vi "Emi EEp.vi"(6 "Num Emi In":u16, 7 "Num Image":u8, 8 "entrée d'erreur":errorcluster caption="entrée d'erreur (pas d'erreur)", 9 "Emi Image EEp":bool, 10 "Matrix en entrée":u8[](array[numeric]), 11 "X-CAN en entrée":refnum<class "X-CAN.lvclass">) -> (0 "sortie d'erreur":errorcluster, 1 "Etat Emi EEp":u16(slide) scale=0.0..512.0, 3 "X-CAN en sortie":refnum<class "X-CAN.lvclass">, 4 "Num Emi Out":u16)   [LabVIEW 2014]
uses:
  <vilib>/Stratom, Inc/X-CAN for myRIO (API)/X-CAN Class/X-CAN.lvclass
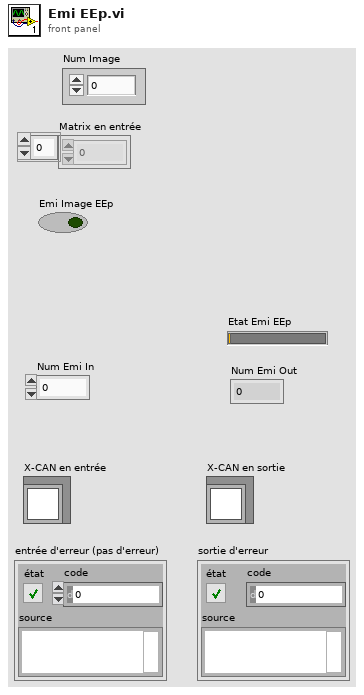
[diagram p1: front panel]
types:
  T1 = cluster{"ID trame":u32, bool, bool, i32[], "seconds since 1Jan1904":timestamp}
  T2 = cluster{"ID trame":u32, bool, bool, u8[], "seconds since 1Jan1904":timestamp}
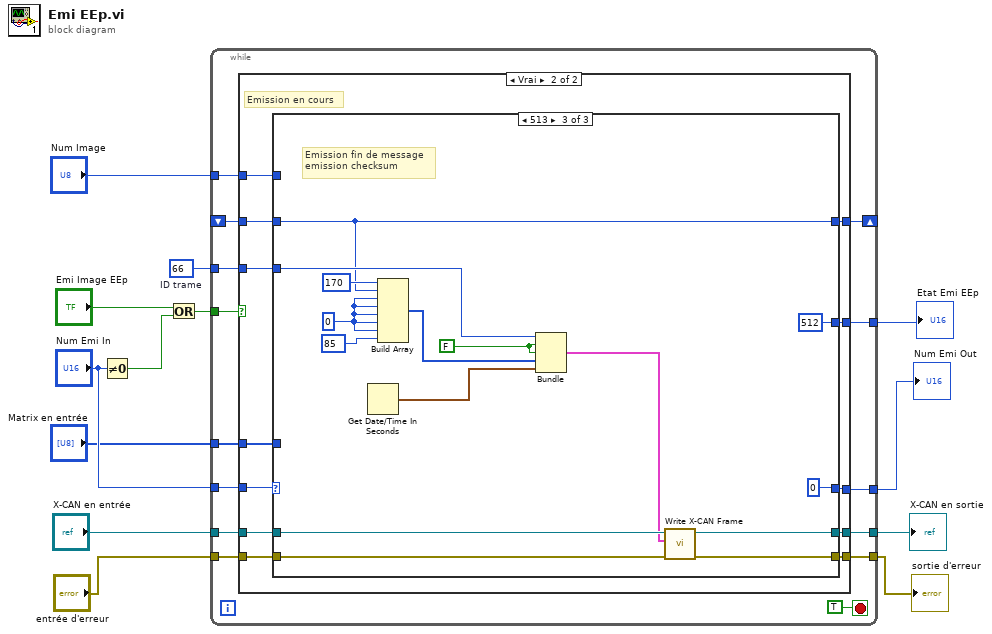
[diagram p0: block diagram]
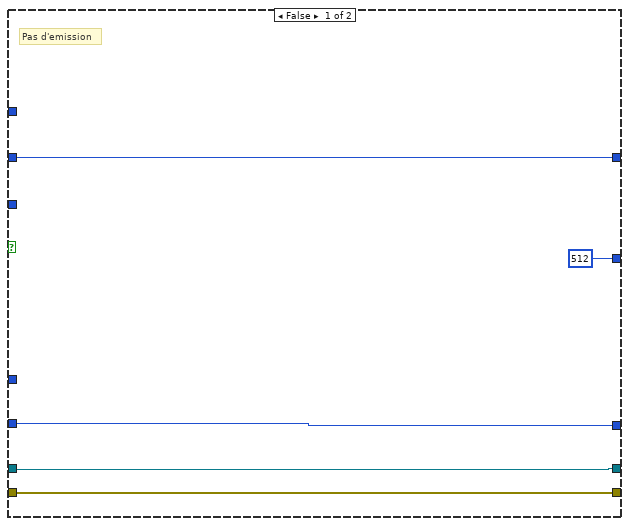
[diagram p2: hidden frame]
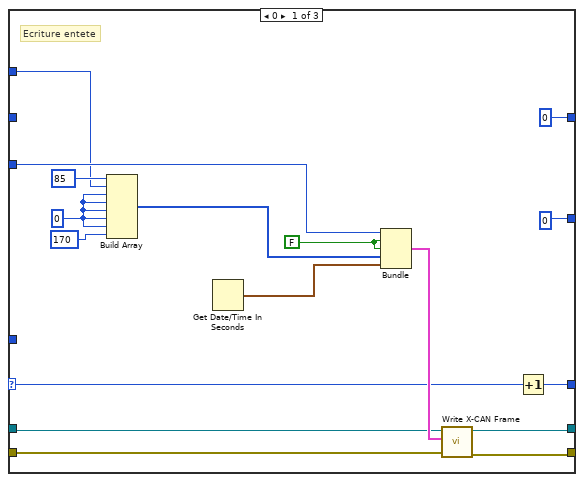
[diagram p3: hidden frame]
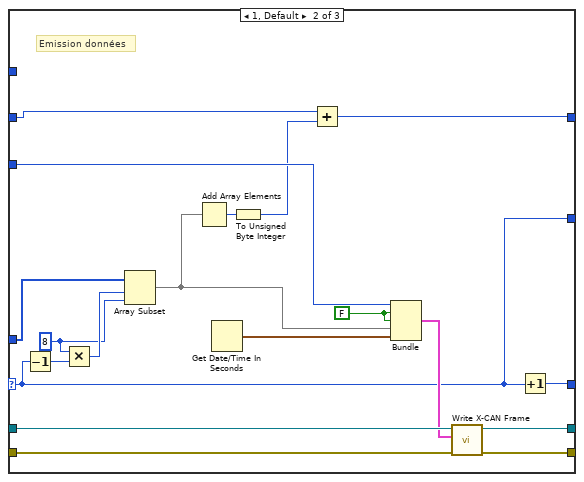
[diagram p4: hidden frame]
diagram:
  w3 = u32 66  # ID trame
  n1 = Not Equal To 0?(x="Num Emi In") -> (x != 0?=w7:bool)
  n2 = Or(x="Emi Image EEp", y=w7) -> (x .or. y?=w9:bool)
  n3 = while {
    tunnel: w9 -> [w23]
    tunnel: "Num Emi In" -> [w22]
    tunnel: [w21] -> w5
    tunnel: [w20] -> w4
    tunnel: w3 -> [w19]
    tunnel: "Matrix en entrée" -> [w18]
    tunnel: "X-CAN en entrée" -> [w24]
    tunnel: [w25] -> w11
    tunnel: "entrée d'erreur" -> [w26]
    tunnel: [w27] -> w13
    shift-right: [w15] -> _
    shift-left: _ -> [w17]
    tunnel: "Num Image" -> [w14]
    stop <- TRUE stop-if-true
    n4 = case shown="Vrai" w23 {
      tunnel: [w32 w44] -> w27
      tunnel: w26 -> [w32 w43]
      tunnel: [w31 w42] -> w25
      tunnel: w24 -> [w31 w41]
      tunnel: w22 -> [w30 w40]
      tunnel: [w30 w39] -> w21
      tunnel: [u16 512 w38] -> w20
      tunnel: w19 -> [_ w37]
      tunnel: w18 -> [_ w36]
      tunnel: w17 -> [w28 w35]
      tunnel: [w28 w34] -> w15
      tunnel: w14 -> [_ w33]
      frame False {
        # "Pas d'emission"
      }
      frame True {
        # "Emission en cours"
        n5 = case shown="513" w40 {
          selector: w40 -> [w50 w67 _]
          tunnel: [w59 w80 w86] -> w44
          tunnel: w43 -> [w57 w79 w87]
          tunnel: [w60 w78 w85] -> w42
          tunnel: w41 -> [w58 w77 w88]
          tunnel: [w51 w71 0] -> w39
          tunnel: [0 w67 512] -> w38
          tunnel: w37 -> [w47 w74 w89]
          tunnel: w36 -> [_ w72 _]
          tunnel: w35 -> [_ w66 w81]
          tunnel: [u8 0 w65 w81] -> w34
          tunnel: w33 -> [w45 _ _]
          frame 0 {
            w48 = 0
            w55 = FALSE
            # "Ecriture entete"
            n6 = Build Array(85, w45, w48, w48, w48, w48, w48, 170) -> (w54:i32[])
            n7 = Get Date/Time In Seconds() -> (seconds since 1Jan1904=w56:timestamp)
            n8 = Bundle("ID trame"=w47, w55, w55, w54, "seconds since 1Jan1904"=w56) -> (w61:T1)  [unwired: 1 in]
            n9 = call <vilib>:"Write X-CAN Frame.vi"("error in"=w57, "CAN Frame"=w61, "X-CAN Session in"=w58) -> ("error out"=w59:errorcluster, "X-CAN Session out"=w60:refnum<class "X-CAN.lvclass">)  [unwired: 7 in]
            n10 = Increment(x=w50) -> (x+1=w51:u16)
          }
          frame 1, Default {
            w68 = u16 8
            w73 = FALSE
            # "Emission données"
            n11 = Decrement(x=w67) -> (x-1=w70:u16)
            n12 = Multiply(x=w68, y=w70) -> (x*y=w69:u16)
            n13 = Array Subset(array=w72, index=w69, length=w68) -> (w64:u8[])
            n14 = Add Array Elements(numeric array=w64) -> (sum=w63:u8)
            n15 = Get Date/Time In Seconds() -> (seconds since 1Jan1904=w75:timestamp)
            n16 = To Unsigned Byte Integer(number=w63) -> (unsigned 8bit integer=w62:u8)
            n17 = Add(x=w66, y=w62) -> (x+y=w65:u8)
            n18 = Bundle("ID trame"=w74, w73, w73, w64, "seconds since 1Jan1904"=w75) -> (w76:T2)  [unwired: 1 in]
            n19 = call <vilib>:"Write X-CAN Frame.vi"("error in"=w79, "CAN Frame"=w76, "X-CAN Session in"=w77) -> ("error out"=w80:errorcluster, "X-CAN Session out"=w78:refnum<class "X-CAN.lvclass">)  [unwired: 7 in]
            n20 = Increment(x=w67) -> (x+1=w71:u16)
          }
          frame 513 {
            w95 = 0
            w91 = FALSE
            # "Emission fin de message\nemission checksum"
            n21 = Get Date/Time In Seconds() -> (seconds since 1Jan1904=w90:timestamp)
            n22 = Build Array(170, w81, w95, w95, w95, w95, w95, 85) -> (w92:i32[])
            n23 = Bundle("ID trame"=w89, w91, w91, w92, "seconds since 1Jan1904"=w90) -> (w84:T1)  [unwired: 1 in]
            n24 = call <vilib>:"Write X-CAN Frame.vi"("error in"=w87, "CAN Frame"=w84, "X-CAN Session in"=w88) -> ("error out"=w86:errorcluster, "X-CAN Session out"=w85:refnum<class "X-CAN.lvclass">)  [unwired: 7 in]
          }
        }
      }
    }
  }
  "Etat Emi EEp" <- w4
  "sortie d'erreur" <- w13
  "X-CAN en sortie" <- w11
  "Num Emi Out" <- w5
